vi "Execute.vi"(5 "Init user event out":refnum<user-event>, 7 "user event in":refnum<user-event>, 8 "Advanced Waveform In":refnum<class "Advanced Waveform.lvclass">, 9 "Message in":refnum<class "Message.lvclass">, 10 "Command Queue":refnum<queue>, 11 "error in (no error)":errorcluster) -> (0 "Advanced Waveform Out":refnum<class "Advanced Waveform.lvclass">, 1 "Message out":refnum<class "Message.lvclass">, 2 "Stop":bool, 3 "error out":errorcluster)   [LabVIEW 2011, in "Message.lvclass"]
uses:
  Message.lvclass
  Advanced Waveform Class/Advanced Waveform.lvclass
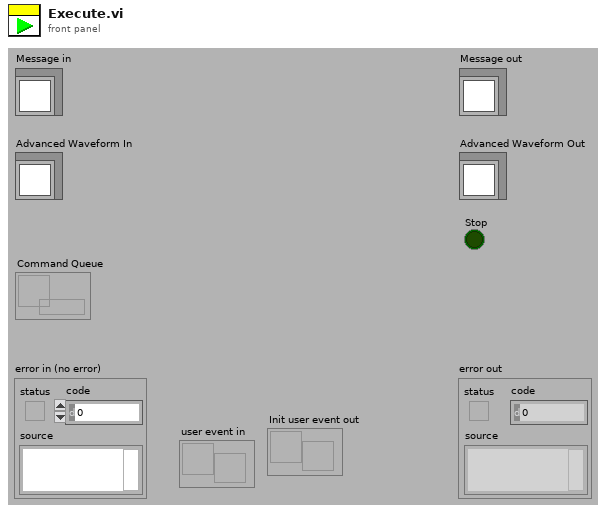
[diagram p1: front panel]
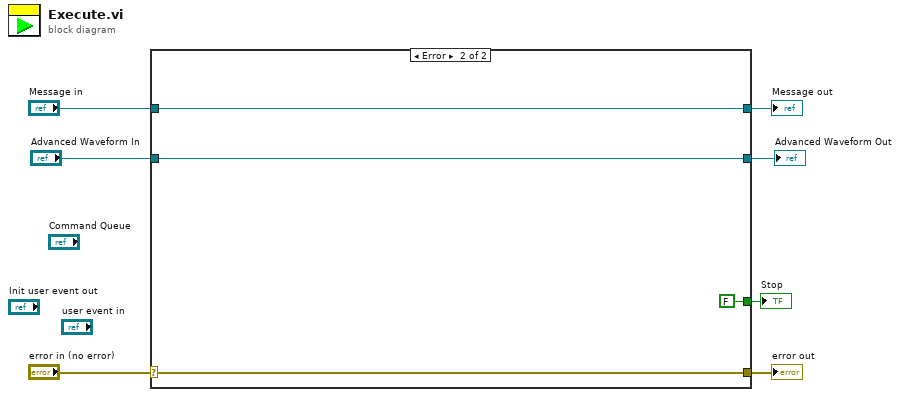
[diagram p0: block diagram]
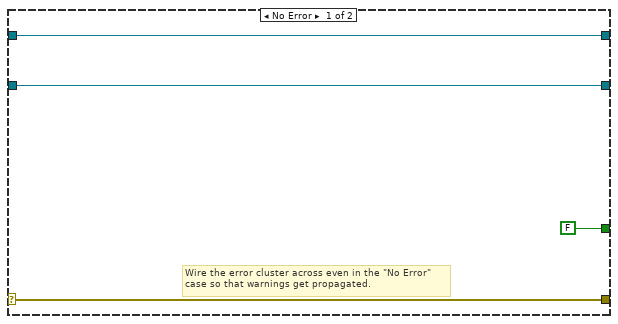
[diagram p2: hidden frame]
diagram:
  n1 = case shown="Error" "error in (no error)" {
    selector: "error in (no error)" -> [w10 w15]
    tunnel: [w10 w15] -> w6
    tunnel: [w11 w14] -> w4
    tunnel: "Message in" -> [w11 w14]
    tunnel: [FALSE FALSE] -> w3
    tunnel: [w8 w12] -> w2
    tunnel: "Advanced Waveform In" -> [w8 w12]
    frame No Error {
      # "Wire the error cluster across even in the \"No Error\"\ncase so that warnings get propagated."
    }
    frame Error {
    }
  }
  "error out" <- w6
  "Message out" <- w4
  "Stop" <- w3
  "Advanced Waveform Out" <- w2
